vi "Get All.vi"(6 "Entity Manager in":refnum<class "Entity Manager.lvclass">, 11 "Entity Collection in":refnum<class "Entity Collection.lvclass">) -> (1 "error out":errorcluster, 2 "Entities":refnum<class "Entity.lvclass">[](array[class]), 3 "Entity Collection":refnum<class "Entity Collection.lvclass">, 4 "Entity Manager":refnum<class "Entity Manager.lvclass">)   [LabVIEW 2020, in "Conditum.lvlib" / "Columns.lvlib" / "Entity Collection.lvclass"]
uses:
  Entity Collection.lvclass
  Entity/Entity.lvclass
  Entity Manager/Entity Manager.lvclass
  Entity Collection.lvclass/Entity Collection.ctl
  Entity/Entity.lvclass/Entity.ctl
  ID/ID.lvclass/ID.ctl
  Entity Manager/Entity Manager.lvclass/Entity Manager.ctl
  ID/Get.vi
  Entity Manager/Check Unit of Work.vi
  Entity Manager/Get or Register Entity.vi
  Unit Of Work Session/Find Entity by ID.vi
  <vilib>/Comparison/Less/Less Functor/Less Functor.lvclass
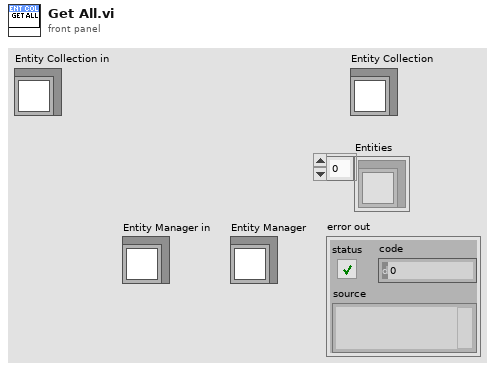
[diagram p1: front panel]
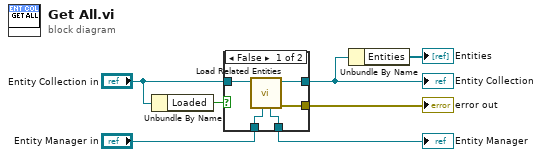
[diagram p0: block diagram]
diagram:
  n1 = Unbundle By Name("Entity Collection in") -> ("Loaded"=w5:bool)
  n2 = case shown="False" w5 {
    tunnel: [w10 w14] -> w4
    tunnel: [w11 w13] -> w7
    tunnel: "Entity Collection in" -> [w12 w14]
    tunnel: [w9 _] -> w1
    tunnel: "Entity Manager in" -> [w8 w13]
    frame False {
      n3 = call "Load Related Entities.vi"("Entity Manager in"=w8, "Entity Collection in"=w12) -> ("error out"=w9:errorcluster, "Entity Collection out"=w10:refnum<class "Entity Collection.lvclass">, "Entity Manager"=w11:refnum<class "Entity Manager.lvclass">)  [unwired: 7 in]
    }
    frame True {
    }
  }
  "Entity Collection" <- w4
  "error out" <- w1
  "Entity Manager" <- w7
  n4 = Unbundle By Name(w4) -> ("Entities"=→"Entities":refnum<class "Entity.lvclass">[])
